vi "Test Event Gloabl.vi"(8 "error in (no error)":errorcluster, 10 "Set (F)":bool, 11 "Test Event in":T1) -> (0 "error out":errorcluster, 1 "Is Set?":bool, 2 "Succeeded?":bool, 3 "Test Event out":T1)   [LabVIEW 2009, in "Caraya.lvlib" / "Basic Test Manager.lvclass"]
uses:
  Basic Test Manager.lvclass
  Test Result/Test Event.ctl
  Test Result/Test Event Data.ctl
  Test Result/Test Result.lvclass
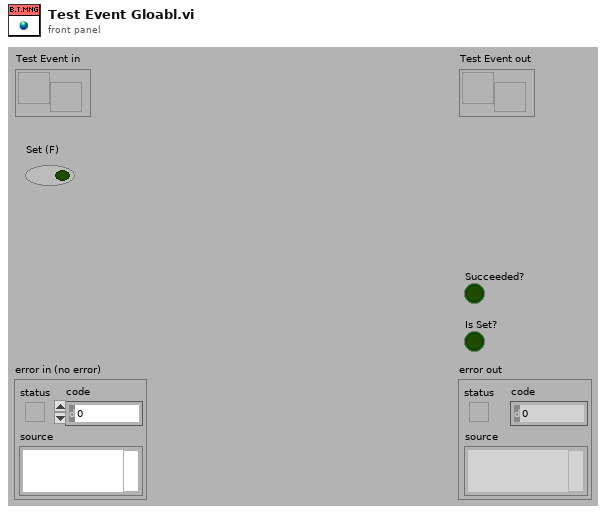
[diagram p1: front panel]
types:
  T1 = typedef "Caraya.lvlib/Test Result.lvclass/Test Event.ctl" = refnum<user-event>
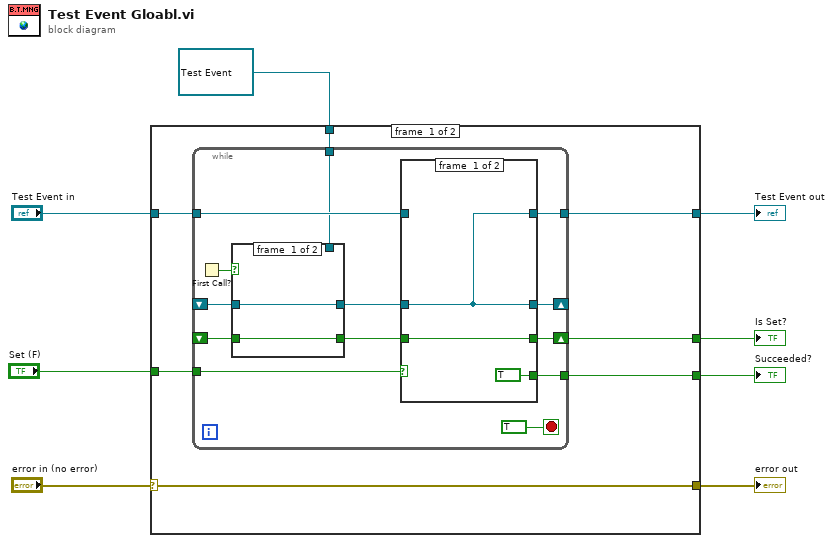
[diagram p0: block diagram]
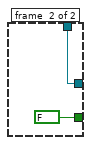
[diagram p2: hidden frame]
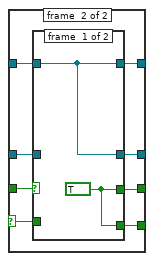
[diagram p3: hidden frame]
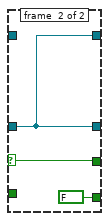
[diagram p4: hidden frame]
diagram:
  n1 = case shown="No Error" "error in (no error)" {
    selector: "error in (no error)" -> [w13 w49]
    tunnel: "Test Event in" -> [w15 w50]
    tunnel: "Set (F)" -> [w14 _]
    tunnel: [w12 w50] -> w5
    tunnel: [w13 w49] -> w4
    tunnel: [w11 _] -> w3
    tunnel: [w10 _] -> w2
    tunnel: T1 refnum ("Test Event in 2") -> [w9 _]
    frame #0 {
      n2 = while {
        tunnel: w14 -> [w27]
        tunnel: w15 -> [w24]
        shift-right: [w22] -> _
        shift-left: _ -> [w25]
        tunnel: [w21] -> w12
        shift-right: [w19] -> w11
        shift-left: _ -> [w20]
        tunnel: [w17] -> w10
        tunnel: w9 -> [w16]
        stop <- TRUE stop-if-true
        n3 = First Call?() -> (First Call?: T/F=w26:bool)
        n4 = case shown="False" w26 {
          tunnel: w25 -> [w30 _]
          tunnel: [w30 w31] -> w23
          tunnel: w20 -> [w29 _]
          tunnel: [w29 FALSE] -> w18
          tunnel: w16 -> [_ w31]
          frame #0 {
          }
          frame #1 {
          }
        }
        n5 = case shown="True" w27 {
          selector: w27 -> [_ w37]
          tunnel: w24 -> [_ w43]
          tunnel: w23 -> [w35 w40]
          tunnel: [w35 w39] -> w22
          tunnel: [w35 w41] -> w21
          tunnel: [w34 w38] -> w19
          tunnel: w18 -> [w34 w42]
          tunnel: [TRUE w36] -> w17
          frame #0 {
          }
          frame #1 {
            n6 = case shown="True" w42 {
              selector: w42 -> [_ w47]
              tunnel: w43 -> [w45 _]
              tunnel: [w45 w48] -> w41
              tunnel: w40 -> [_ w48]
              tunnel: [w45 w48] -> w39
              tunnel: [w44 w47] -> w38
              tunnel: w37 -> [_ _]
              tunnel: [w44 FALSE] -> w36
              frame #0 {
                w44 = TRUE
              }
              frame #1 {
              }
            }
          }
        }
      }
    }
    frame #1 {
    }
  }
  "error out" <- w4
  "Test Event out" <- w5
  "Is Set?" <- w3
  "Succeeded?" <- w2
